vi "ReversedEngineering TypeDefToClass.vi"(1 "TypeDef":T7) -> (15 "NodeClassInfo":T1)   [LabVIEW 2012]
uses:
  <resource>/Framework/Providers/Open_GDS/UML/ReversedEngineering/ReversedEngineering TypeDefType.ctl
  <resource>/Framework/Providers/Open_GDS/UML/ReversedEngineering/ReversedEngineering AttributeInfoType.ctl
  <resource>/Framework/Providers/Open_GDS/ClassProviders/Common/CommonVIs/CommonVIs_AttributeDataType.ctl
  <resource>/Framework/Providers/Open_GDS/UML/UMLEditor/UMLEditor_VisibilityType.ctl
  <resource>/Framework/Providers/Open_GDS/UML/ReversedEngineering/ReversedEngineering ClassInfoType.ctl
  <resource>/Framework/Providers/Open_GDS/UML/ReversedEngineering/ReversedEngineering_ClassDependencyDetailsType.ctl
  <resource>/Framework/Providers/Open_GDS/ClassProviders/Common/ScriptingFunctions/SubVIs/Scripting_ViDependencyType.ctl
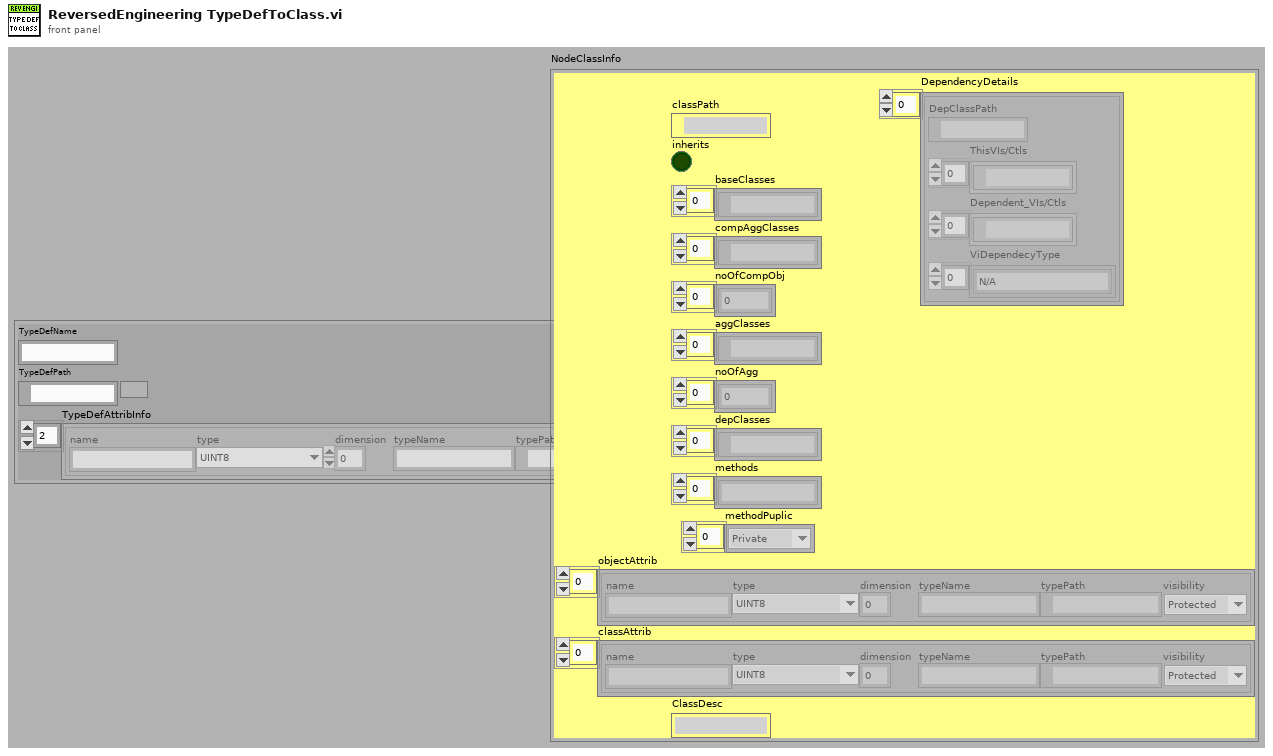
[diagram p1: front panel]
types:
  T1 = typedef "ReversedEngineering ClassInfoType.ctl" = cluster{"classPath":path, "inherits":bool, "baseClasses":path[], "compAggClasses":path[], "noOfCompObj":i32[], "aggClasses":path[], "noOfAgg":i32[], "depClasses":path[], "methods":string[], "methodPuplic":T2[], "objectAttrib":T3[], "classAttrib":T3[], "ClassDesc":string, "DependencyDetails":T5[]}
  T2 = typedef "UMLEditor_VisibilityType.ctl" = enum16{"Public", "Private", "Protected"}
  T3 = typedef "ReversedEngineering AttributeInfoType.ctl" = cluster{"name":string, "type":T4, "dimension":i32, "typeName":string, "typePath":path, "visibility":T2}
  T4 = typedef "CommonVIs_AttributeDataType.ctl" = enum16{"UINT8", "INT8", "UINT16", "INT16", "UINT32", "INT32", "UINT64", "INT64", "SGL", "DBL", "EXT", "CSG", "CDB", "CXT", "TimeStamp", "STRING", "PATH", "BOOL", "ENUM", "RefNum", "VIRefNum", "LabVIEW Class", "Cluster", "Variant", "TypeDef", "Waveform", "LabVIEW Object", "Other"}
  T5 = typedef "ReversedEngineering_ClassDependencyDetailsType.ctl" = cluster{"DepClassPath":path, "ThisVIs/Ctls":path[], "Dependent_VIs/Ctls":path[], "ViDependecyType":T6[]}
  T6 = typedef "Scripting_ViDependencyType.ctl" = enum16{"N/A", "Launches"}
  T7 = typedef "ReversedEngineering TypeDefType.ctl" = cluster{"TypeDefName":string, "TypeDefPath":path, "TypeDefAttribInfo":T3[]}
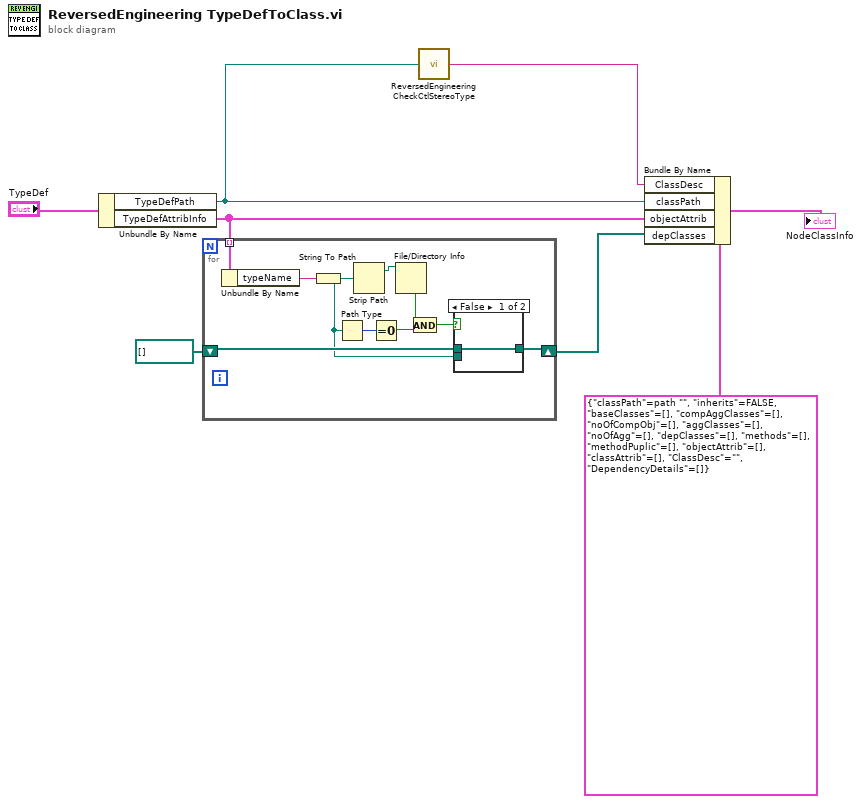
[diagram p0: block diagram]
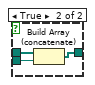
[diagram p2: hidden frame]
diagram:
  n1 = Unbundle By Name("TypeDef") -> ("TypeDefPath"=w1:path, "TypeDefAttribInfo"=w5:T3[])
  n2 = for {
    tunnel: w5 -> [w18] mode=indexing
    shift-right: [w10] -> w3
    shift-left: path[] [] -> [w11]
    n3 = Unbundle By Name(w18) -> ("typeName"=w17:string)
    n4 = String To Path(string=w17) -> (path=w9:path)
    n5 = Path Type(1:w9) -> (0:w16:i16)
    n6 = Strip Path(path=w9) -> (stripped path=w15:path)  [unwired: 1 out]
    n7 = Equal To 0?(x=w16) -> (x = 0?=w14:bool)
    n8 = File/Directory Info(path=w15) -> (directory=w13:bool)  [unwired: 1 in, 6 out]
    n9 = And(x=w13, y=w14) -> (x .and. y?=w12:bool)
    n10 = case shown="False" w12 {
      tunnel: w11 -> [w19 w22]
      tunnel: [w19 w21] -> w10
      tunnel: w9 -> [_ w20]
      frame False {
      }
      frame True {
        n11 = Build Array (concatenate)(w22, w20) -> (w21:path[])
      }
    }
  }
  n12 = call <resource>:"ReversedEngineering CheckCtlStereoType.vi"("TypeDefPath"=w1) -> ("ClassDesc"=w2:string)
  n13 = Bundle By Name(cluster=T1 {"classPath"=path "", "inherits"=FALSE, "baseClasses"=[], "compAggClasses"=[], "noOfCompObj"=[], "aggClasses"=[], "noOfAgg"=[], "depClasses"=[], "methods"=[], "methodPuplic"=[], "objectAttrib"=[], "classAttrib"=[], "ClassDesc"="", "DependencyDetails"=[]} ("classInfo"), "ClassDesc"=w2, "classPath"=w1, "objectAttrib"=w5, "depClasses"=w3) -> (→"NodeClassInfo":T1)
